vi "Write version.vi"(8 "error in (no error)":errorcluster, 10 "Version":i32, 11 "CoSy Config File in":refnum<class "CoSy Config File.lvclass">) -> (0 "error out":errorcluster, 3 "CoSy Config File out":refnum<class "CoSy Config File.lvclass">)   [LabVIEW 2011, in "COSYLib.lvlib" / "CoSy Config File.lvclass"]
doc: "Returns the version of the configuration file, as specified in the \"version\" attribute of the root tag.\n\nReturns a number; if the version has an invalid value, a version of \"-1\" is returned."
uses:
  CoSy Config File.lvclass
  CoSy Config File.lvclass/CoSy Config File.ctl
  <vilib>/xml/Close Reference(NNMap).vi
  <vilib>/xml/Close Reference(Node).vi
  <vilib>/xml/NI_XML.lvlib
  C:/Program Files (x86)/National Instruments/LabVIEW 2011/resource/objmgr/DOMUserDefRef.rc
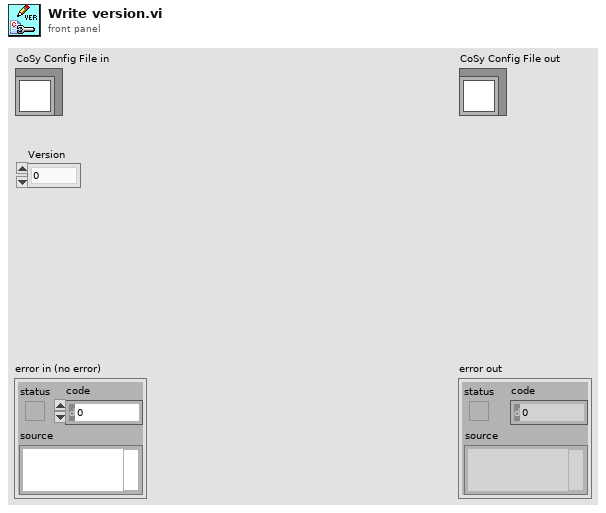
[diagram p1: front panel]
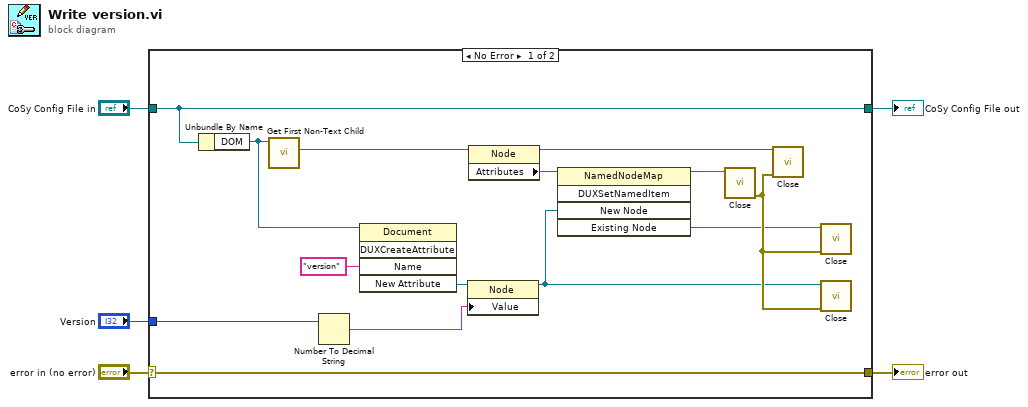
[diagram p0: block diagram]
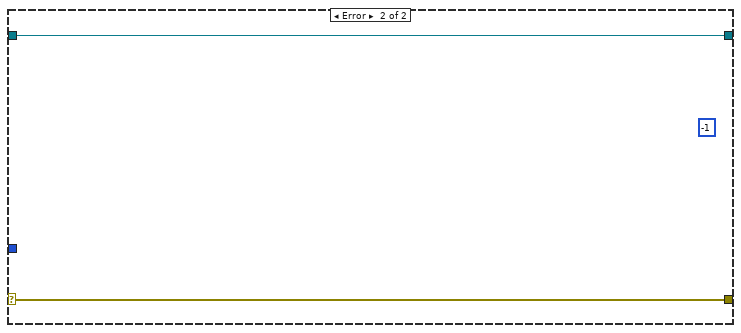
[diagram p2: hidden frame]
diagram:
  n1 = case shown="No Error" "error in (no error)" {
    selector: "error in (no error)" -> [w19 w21]
    tunnel: [w19 w21] -> w4
    tunnel: [w17 w20] -> w2
    tunnel: "CoSy Config File in" -> [w17 w20]
    tunnel: "Version" -> [w11 _]
    frame No Error {
      n2 = Unbundle By Name(w17) -> ("DOM"=w14:refnum<k20>)
      n3 = call <vilib>:"Get First Non-Text Child.vi"("node in"=w14) -> ("child node"=w15:refnum<k20>)  [unwired: 7 in, 3 out]
      n4 = Number To Decimal String(number=w11) -> (decimal integer string=w10:string)  [unwired: 1 in]
      n5 = invoke class="Document" method="DUXCreateAttribute"(reference=w14, "Name"="version" ("Attribute name")) -> ("New Attribute"=w12:refnum<k20>)  [unwired: 3 in, 4 out]
      n6 = property class="Node"(reference=w12, "Value"=w10) -> (reference out=w9:refnum<k20>)  [unwired: 1 in, 1 out]
      n7 = property class="Node"(reference=w15) -> (reference out=w6:refnum<k20>, "Attributes"=w16:refnum<k20>)  [unwired: 1 in, 1 out]
      n8 = invoke class="NamedNodeMap" method="DUXSetNamedItem"(reference=w16, "New Node"=w9) -> (reference out=w7:refnum<k20>, "Existing Node"=w8:refnum<k20>)  [unwired: 3 in, 3 out]
      n9 = call-poly <vilib>:"Close.vi"("named node map"=w7) -> ("error out"=w18:errorcluster)  [unwired: 8 in]
      n10 = call-poly <vilib>:"Close.vi"("error in (no error)"=w18, "node"=w6) -> ()  [unwired: 7 in, 1 out]
      n11 = call-poly <vilib>:"Close.vi"("error in (no error)"=w18, "node"=w8) -> ()  [unwired: 7 in, 1 out]
      n12 = call-poly <vilib>:"Close.vi"("error in (no error)"=w18, "node"=w9) -> ()  [unwired: 7 in, 1 out]
    }
    frame Error {
      (unwired) -1
    }
  }
  "error out" <- w4
  "CoSy Config File out" <- w2
